vi "Motor Delay subvi.vi"(0 "Y axis":dbl, 1 "Button":bool, 2 "X axis":dbl) -> ()   [LabVIEW 2013]
uses:
  Training codes/Global X axis.vi
  2-19/Global Y axis.vi
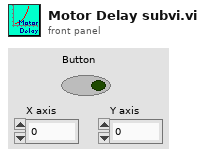
[diagram p1: front panel]
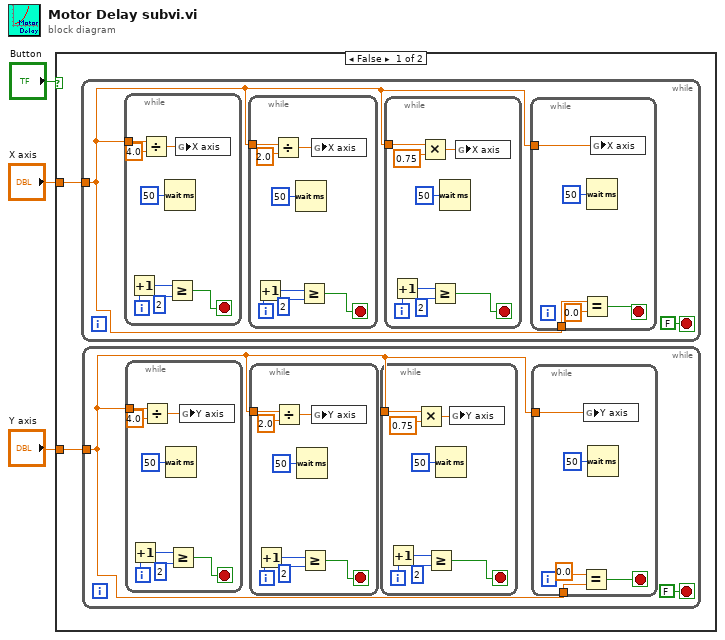
[diagram p0: block diagram]
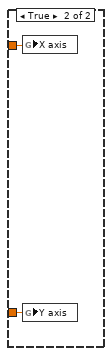
[diagram p2: hidden frame]
diagram:
  n1 = case shown="False" "Button" {
    tunnel: "X axis" -> [w4 w68]
    tunnel: "Y axis" -> [w5 w69]
    frame False {
      n2 = while {
        tunnel: w4 -> [w38]
        stop <- FALSE stop-if-true
        n3 = while {
          tunnel: w38 -> [w67]
          i -> [w64]
          stop <- w60 stop-if-true
          n4 = Increment(x=w64) -> (x+1=w63:i32)
          n5 = Divide(x=w67, y=4.0) -> (x/y=w66:dbl)
          n6 = Wait (ms)(milliseconds to wait=50) -> ()  [unwired: 1 out]
          n7 = Greater Or Equal?(x=w63, y=2) -> (x >= y?=w60:bool)
          n8 = global write "Global X axis.vi" "X axis"(w66) -> ()
        }
        n9 = while {
          tunnel: w38 -> [w59]
          i -> [w53]
          stop <- w52 stop-if-true
          n10 = Increment(x=w53) -> (x+1=w54:i32)
          n11 = Divide(x=w59, y=2.0) -> (x/y=w58:dbl)
          n12 = Wait (ms)(milliseconds to wait=50) -> ()  [unwired: 1 out]
          n13 = Greater Or Equal?(x=w54, y=2) -> (x >= y?=w52:bool)
          n14 = global write "Global X axis.vi" "X axis"(w58) -> ()
        }
        n15 = while {
          tunnel: w38 -> [w51]
          i -> [w44]
          stop <- w45 stop-if-true
          n16 = Increment(x=w44) -> (x+1=w48:i32)
          n17 = Multiply(x=w51, y=0.75) -> (x*y=w50:dbl)
          n18 = Greater Or Equal?(x=w48, y=2) -> (x >= y?=w45:bool)
          n19 = Wait (ms)(milliseconds to wait=50) -> ()  [unwired: 1 out]
          n20 = global write "Global X axis.vi" "X axis"(w50) -> ()
        }
        n21 = while {
          tunnel: w38 -> [w43]
          tunnel: w38 -> [w39]
          stop <- w40 stop-if-true
          n22 = Equal?(x=w39, y=0.0) -> (x = y?=w40:bool)
          n23 = Wait (ms)(milliseconds to wait=50) -> ()  [unwired: 1 out]
          n24 = global write "Global X axis.vi" "X axis"(w43) -> ()
        }
      }
      n25 = while {
        tunnel: w5 -> [w7]
        stop <- FALSE stop-if-true
        n26 = while {
          tunnel: w7 -> [w36]
          i -> [w34]
          stop <- w30 stop-if-true
          n27 = Increment(x=w34) -> (x+1=w33:i32)
          n28 = Divide(x=w36, y=4.0) -> (x/y=w29:dbl)
          n29 = Wait (ms)(milliseconds to wait=50) -> ()  [unwired: 1 out]
          n30 = Greater Or Equal?(x=w33, y=2) -> (x >= y?=w30:bool)
          n31 = global write "Global Y axis.vi" "Y axis"(w29) -> ()
        }
        n32 = while {
          tunnel: w7 -> [w28]
          i -> [w23]
          stop <- w22 stop-if-true
          n33 = Increment(x=w23) -> (x+1=w24:i32)
          n34 = Divide(x=w28, y=2.0) -> (x/y=w21:dbl)
          n35 = Wait (ms)(milliseconds to wait=50) -> ()  [unwired: 1 out]
          n36 = Greater Or Equal?(x=w24, y=2) -> (x >= y?=w22:bool)
          n37 = global write "Global Y axis.vi" "Y axis"(w21) -> ()
        }
        n38 = while {
          tunnel: w7 -> [w20]
          i -> [w14]
          stop <- w15 stop-if-true
          n39 = Increment(x=w14) -> (x+1=w18:i32)
          n40 = Multiply(x=w20, y=0.75) -> (x*y=w13:dbl)
          n41 = Greater Or Equal?(x=w18, y=2) -> (x >= y?=w15:bool)
          n42 = Wait (ms)(milliseconds to wait=50) -> ()  [unwired: 1 out]
          n43 = global write "Global Y axis.vi" "Y axis"(w13) -> ()
        }
        n44 = while {
          tunnel: w7 -> [w11]
          tunnel: w7 -> [w9]
          stop <- w8 stop-if-true
          n45 = Equal?(x=0.0, y=w9) -> (x = y?=w8:bool)
          n46 = global write "Global Y axis.vi" "Y axis"(w11) -> ()
          n47 = Wait (ms)(milliseconds to wait=50) -> ()  [unwired: 1 out]
        }
      }
    }
    frame True {
      n48 = global write "Global X axis.vi" "X axis"(w68) -> ()
      n49 = global write "Global Y axis.vi" "Y axis"(w69) -> ()
    }
  }
